vi "Play Next Turn.vi"(4 "Player 2 Score":i64, 6 "Player 1 Score":i64, 7 "Player 1 Turn?":bool, 8 "Player 2 Position":i64, 9 "Player 1 Position":i64) -> (2 "Player 2 Wins Out":i64, 3 "Player 1 Wins Out":i64)   [LabVIEW 2021]
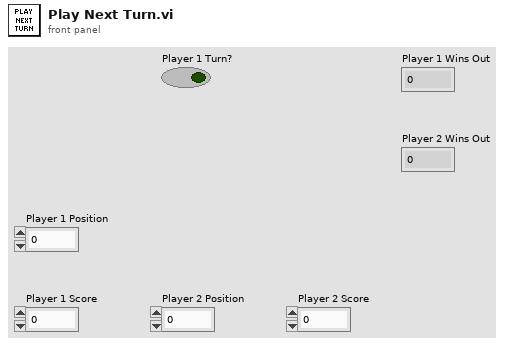
[diagram p1: front panel]
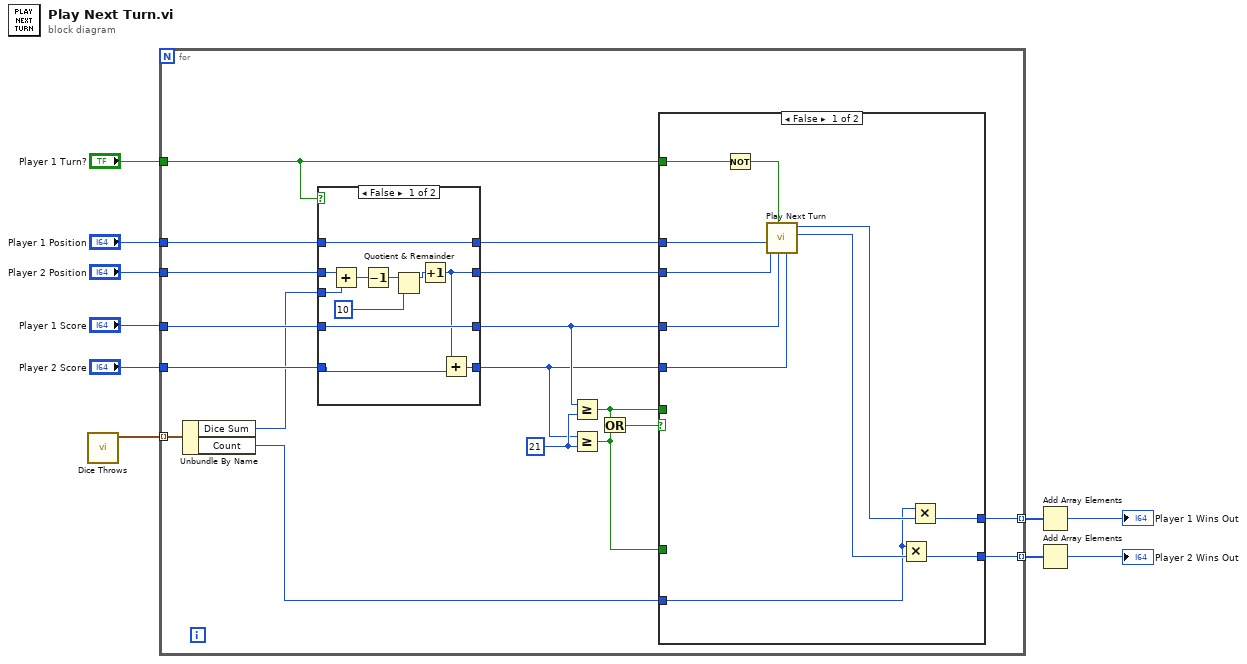
[diagram p0: block diagram]
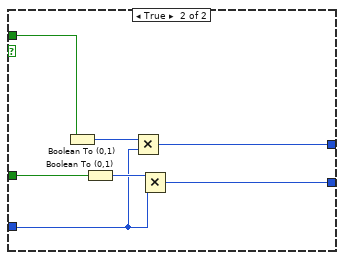
[diagram p2: hidden frame]
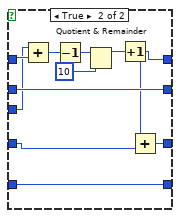
[diagram p3: hidden frame]
diagram:
  n1 = call "Dice Throws.vi"() -> ("Dice Out"=w3:cluster{"Dice Sum":i64, "Count":i64}[])  [unwired: 11 in]
  n2 = for {
    tunnel: w3 -> [w22] mode=indexing
    tunnel: "Player 1 Turn?" -> [w13]
    tunnel: [w24] -> w9 mode=indexing
    tunnel: [w23] -> w10 mode=indexing
    tunnel: "Player 1 Position" -> [w28]
    tunnel: "Player 2 Position" -> [w27]
    tunnel: "Player 1 Score" -> [w26]
    tunnel: "Player 2 Score" -> [w25]
    w21 = i64 21 ("y")
    n3 = Unbundle By Name(w22) -> ("Dice Sum"=w18:i64, "Count"=w16:i64)
    n4 = case shown="False" w13 {
      tunnel: w28 -> [w57 w67]
      tunnel: w27 -> [w52 w68]
      tunnel: [w47 w68] -> w14
      tunnel: [w57 w58] -> w15
      tunnel: w18 -> [w51 w66]
      tunnel: w26 -> [w56 w59]
      tunnel: w25 -> [w49 w65]
      tunnel: [w50 w65] -> w11
      tunnel: [w56 w60] -> w12
      frame False {
        n5 = Add(x=w52, y=w51) -> (x+y=w55:i64)
        n6 = Decrement(x=w55) -> (x-1=w54:i64)
        n7 = Quotient & Remainder(x=w54, y=i64 10) -> (x-y*floor(x/y)=w53:i64)  [unwired: 1 out]
        n8 = Increment(x=w53) -> (x+1=w47:i64)
        n9 = Add(x=w47, y=w49) -> (x+y=w50:i64)
      }
      frame True {
        n10 = Add(x=w66, y=w67) -> (x+y=w64:i64)
        n11 = Decrement(x=w64) -> (x-1=w63:i64)
        n12 = Quotient & Remainder(x=w63, y=i64 10) -> (x-y*floor(x/y)=w61:i64)  [unwired: 1 out]
        n13 = Increment(x=w61) -> (x+1=w58:i64)
        n14 = Add(x=w58, y=w59) -> (x+y=w60:i64)
      }
    }
    n15 = Greater Or Equal?(x=w12, y=w21) -> (x >= y?=w20:bool)
    n16 = Greater Or Equal?(x=w11, y=w21) -> (x >= y?=w19:bool)
    n17 = Or(x=w20, y=w19) -> (x .or. y?=w17:bool)
    n18 = case shown="False" w17 {
      tunnel: [w31 w41] -> w24
      tunnel: [w30 w40] -> w23
      tunnel: w20 -> [_ w46]
      tunnel: w19 -> [_ w45]
      tunnel: w16 -> [w29 w42]
      tunnel: w15 -> [w39 _]
      tunnel: w14 -> [w32 _]
      tunnel: w13 -> [w38 _]
      tunnel: w12 -> [w36 _]
      tunnel: w11 -> [w35 _]
      frame False {
        n19 = Not(x=w38) -> (.not. x?=w37:bool)
        n20 = call "Play Next Turn.vi"("Player 2 Score"=w35, "Player 1 Score"=w36, "Player 1 Turn?"=w37, "Player 2 Position"=w32, "Player 1 Position"=w39) -> ("Player 2 Wins Out"=w33:i64, "Player 1 Wins Out"=w34:i64)  [unwired: 5 in]
        n21 = Multiply(x=w29, y=w33) -> (x*y=w30:i64)
        n22 = Multiply(x=w29, y=w34) -> (x*y=w31:i64)
      }
      frame True {
        n23 = Boolean To (0,1)(Boolean=w46) -> (0, 1=w44:i16)
        n24 = Boolean To (0,1)(Boolean=w45) -> (0, 1=w43:i16)
        n25 = Multiply(x=w44, y=w42) -> (x*y=w41:i64)
        n26 = Multiply(x=w43, y=w42) -> (x*y=w40:i64)
      }
    }
  }
  n27 = Add Array Elements(numeric array=w9) -> (sum=→"Player 1 Wins Out":i64)
  n28 = Add Array Elements(numeric array=w10) -> (sum=→"Player 2 Wins Out":i64)
